vi "IntersectionExample_LV2009.vi"() -> ()   [LabVIEW 2009]
panel:
  in  "Y2 constant value":dbl
  out "Intersection points":dbl[](array[numeric])
  out "X":dbl[](array[numeric])
  out "XY Graph":cluster{dbl[], dbl[]}[](graph)
  out "Y1":dbl[](array[numeric])
  out "Y2":dbl[](array[numeric])
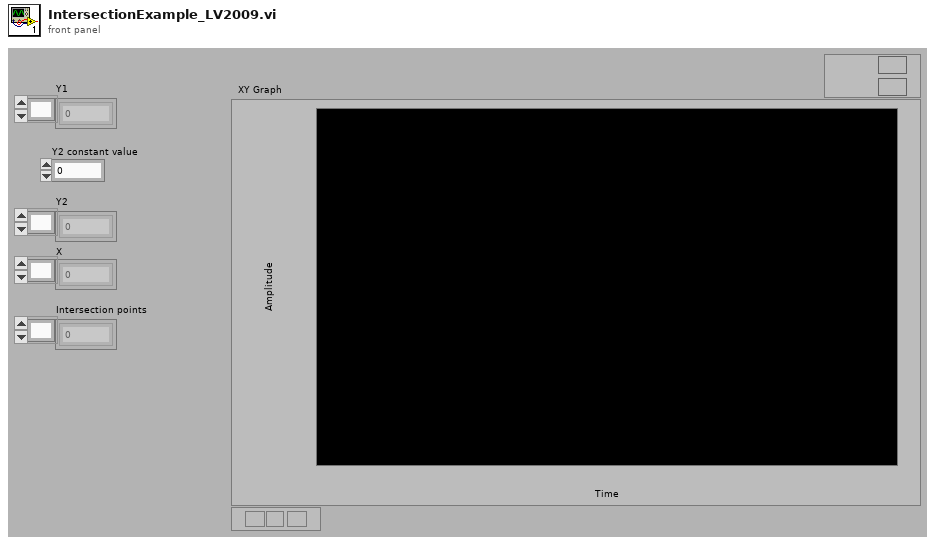
[diagram p1: front panel]
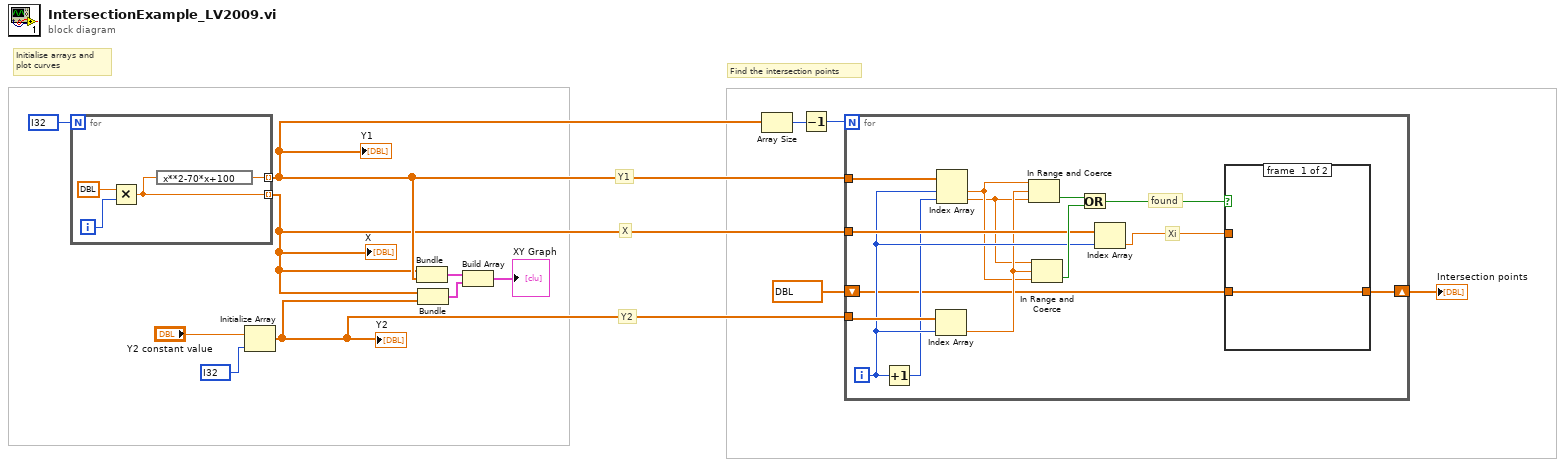
[diagram p0: block diagram]
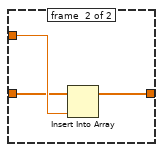
[diagram p2: hidden frame]
diagram:
  # "Y1"
  # "Y2"
  # "X"
  # "Initialise arrays and\nplot curves"
  # "Find the intersection points"
  n1 = for {
    N: i32 ? -> [_]
    tunnel: [w17] -> w8 mode=indexing
    tunnel: [w14] -> w6 mode=indexing
    i -> [w16]
    n2 = Multiply(x=dbl ?, y=w16) -> (x*y=w14:dbl)
    n3 = expression code="x**2-70*x+100"(w14) -> (w17:dbl)
  }
  "Y1" <- w8
  "X" <- w6
  n4 = Initialize Array("Y2 constant value", i32 ? ("dimension size")) -> (w7:dbl[])
  "Y2" <- w7
  n5 = Bundle(w6, w8) -> (w11:cluster{dbl[], dbl[]})  [unwired: 1 in]
  n6 = Bundle(w6, w7) -> (w10:cluster{dbl[], dbl[]})  [unwired: 1 in]
  n7 = Build Array(w11, w10) -> (→"XY Graph":cluster{dbl[], dbl[]}[])
  n8 = Array Size(array=w8) -> (size(s)=w3:i32)
  n9 = Decrement(x=w3) -> (x-1=w2:i32)
  n10 = for {
    N: w2 -> [_]
    tunnel: w8 -> [w31]
    tunnel: w7 -> [w30]
    tunnel: w6 -> [w27]
    shift-right: [w19] -> w4
    shift-left: dbl[] ? -> [w20]
    i -> [w26]
    # "found"
    # "Xi"
    n11 = Increment(x=w26) -> (x+1=w25:i32)
    n12 = Index Array(array=w30, index=w26) -> (element=w24:dbl)
    n13 = Index Array(array=w31, index #1=w26, index #2=w25) -> (element #1=w23:dbl, element #2=w22:dbl)
    n14 = In Range and Coerce(upper limit=w23, x=w24, lower limit=w22) -> (In Range?=w29:bool)  [unwired: 1 out]
    n15 = In Range and Coerce(upper limit=w22, x=w24, lower limit=w23) -> (In Range?=w28:bool)  [unwired: 1 out]
    n16 = Or(x=w29, y=w28) -> (x .or. y?=w21:bool)
    n17 = Index Array(array=w27, index=w26) -> (element=w18:dbl)
    n18 = case shown="True" w21 {
      tunnel: w18 -> [_ w35]
      tunnel: w20 -> [w32 w34]
      tunnel: [w32 w33] -> w19
      frame #0 {
      }
      frame #1 {
        n19 = Insert Into Array(array=w34, new element=w35) -> (w33:dbl[])  [unwired: 1 in]
      }
    }
  }
  "Intersection points" <- w4
